vi "niRFUtil MEAS Max LO Offset.vi"(8 "Meas2 LO Offset (Hz)":dbl, 9 "Meas2 Sampling Rate (Hz)":dbl, 10 "Meas1 LO Offset (Hz)":dbl, 11 "Meas1 Sampling Rate (Hz)":dbl) -> (3 "Max LO Offset (Hz)":dbl)   [LabVIEW 2015, in "niRFUtil.lvlib"]
uses:
  niRFUtil.lvlib
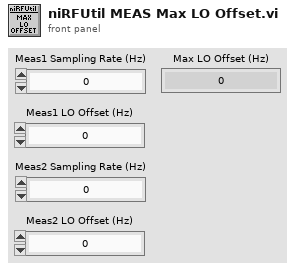
[diagram p1: front panel]
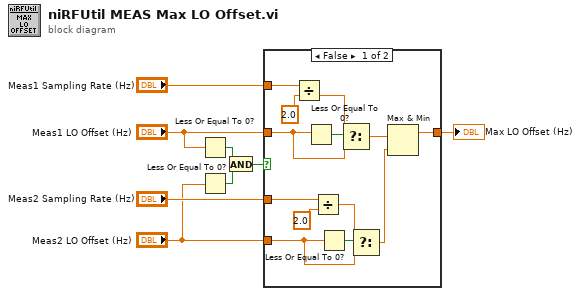
[diagram p0: block diagram]
diagram:
  n1 = Less Or Equal To 0?(x="Meas1 LO Offset (Hz)") -> (x <= 0?=w2:bool)
  n2 = Less Or Equal To 0?(x="Meas2 LO Offset (Hz)") -> (x <= 0?=w1:bool)
  n3 = And(x=w2, y=w1) -> (x .and. y?=w3:bool)
  n4 = case shown="False" w3 {
    tunnel: [w21 w22] -> w8
    tunnel: "Meas2 Sampling Rate (Hz)" -> [w10 _]
    tunnel: "Meas1 Sampling Rate (Hz)" -> [w19 _]
    tunnel: "Meas1 LO Offset (Hz)" -> [w18 w22]
    tunnel: "Meas2 LO Offset (Hz)" -> [w15 _]
    frame False {
      n5 = Divide(x=w19, y=2.0 ("x")) -> (x/y=w13:dbl)
      n6 = Less Or Equal To 0?(x=w18) -> (x <= 0?=w20:bool)
      n7 = Divide(x=w10, y=2.0) -> (x/y=w9:dbl)
      n8 = Less Or Equal To 0?(x=w15) -> (x <= 0?=w16:bool)
      n9 = Select(t=w13, s=w20, f=w18) -> (s? t:f=w17:dbl)
      n10 = Select(t=w9, s=w16, f=w15) -> (s? t:f=w14:dbl)
      n11 = Max & Min(x=w17, y=w14) -> (max(x,y)=w21:dbl)  [unwired: 1 out]
    }
    frame True {
    }
  }
  "Max LO Offset (Hz)" <- w8
